vi "initialization.vi"   [LabVIEW 2016]
doc: "This VI is used to initize the events and flags in the FSM. In the future, it may be used to initize the variables in other function VIs."
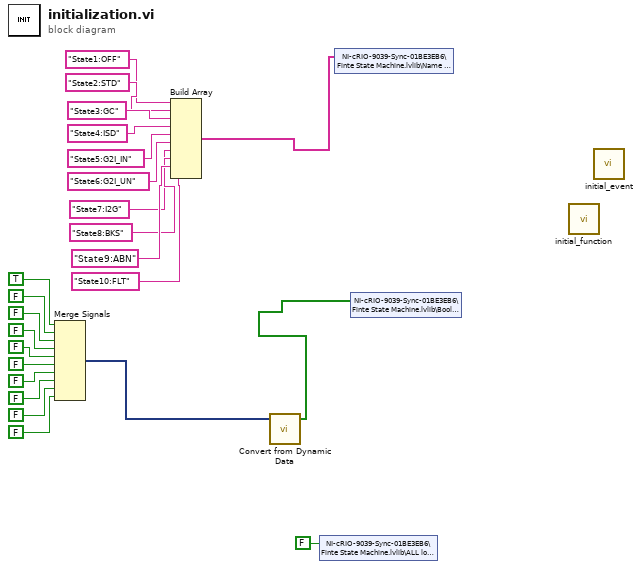
[diagram p0: block diagram]
diagram:
  n1 = Merge Signals(TRUE ("State3"), FALSE ("State3"), FALSE ("State3"), FALSE ("State3"), FALSE ("State3"), FALSE ("State3"), FALSE ("State3"), FALSE ("State3"), FALSE ("State3"), FALSE ("State3")) -> (w14:dynamicdata)
  n2 = Build Array("State1:OFF", "State2:STD", "State3:GC", "State4:ISD", "State5:G2I_IN", "State6:G2I_UN", "State7:I2G", "State8:BKS", "State9:ABN", "State10:FLT") -> (w3:string[])
  n3 = call "Convert from Dynamic Data"("Dynamic Data Type"=w14) -> ("Array"=w2:bool[])  [unwired: 3 in]
  n4 = shared-variable "NI-cRIO-9039-Sync-01BE3EB6\\Finte State Machine.lvlib\\ALL loop stop"(FALSE ("ALL loop stop")) -> ()  [unwired: 1 in, 1 out]
  n5 = shared-variable "NI-cRIO-9039-Sync-01BE3EB6\\Finte State Machine.lvlib\\Name of state"(w3) -> ()  [unwired: 1 in, 1 out]
  n6 = shared-variable "NI-cRIO-9039-Sync-01BE3EB6\\Finte State Machine.lvlib\\Bool of state"(w2) -> ()  [unwired: 1 in, 1 out]
  n7 = call "initial_function.vi"() -> ()  [unwired: 12 in]
  n8 = call "initial_event.vi"() -> ()  [unwired: 12 in]
